vi "FileManager.vi"(6 "Function":enum16{"Switch", "Train"}(ring)=enum."Train", 8 "error in":errorcluster, 11 "file path":path=path "D:/Minecraft/mmc-stable-win32/MultiMC/instances/TRAINS 3-/.minecraft/saves/trains/opencomputers/442cd0d6-e139-46e7-881b-600456d36bc7/home") -> (0 "error out":errorcluster, 1 "SwitchDataArray":T1(array[cluster]), 2 "PathArray":path[](array[path]), 3 "TrainDataArray":T2(array[cluster]), 5 "RootPathArray":path[](array[path]))   [LabVIEW 2014]
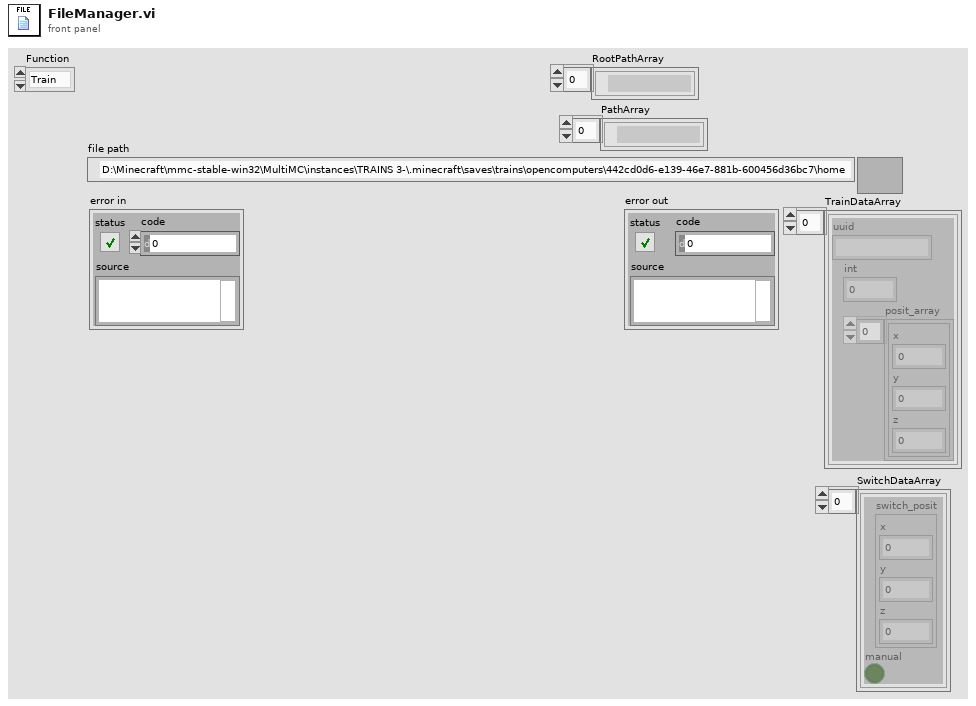
[diagram p1: front panel]
types:
  T1 = cluster{"switch_posit":cluster{"x":dbl, "y":dbl, "z":dbl}, "manual":bool}[]
  T2 = cluster{"uuid":string, "int":i32, "posit_array":cluster{"x":dbl, "y":dbl, "z":dbl}[]}[]
  T3 = cluster{"uuid":string, "int":i32, "posit_array":cluster{"x":dbl, "y":dbl, "z":dbl}[]}
  T4 = enum16{"open", "replace", "create", "open or create", "replace or create", "replace or create with confirmation"}
  T5 = cluster{"switch_posit":cluster{"x":dbl, "y":dbl, "z":dbl}, "manual":bool}
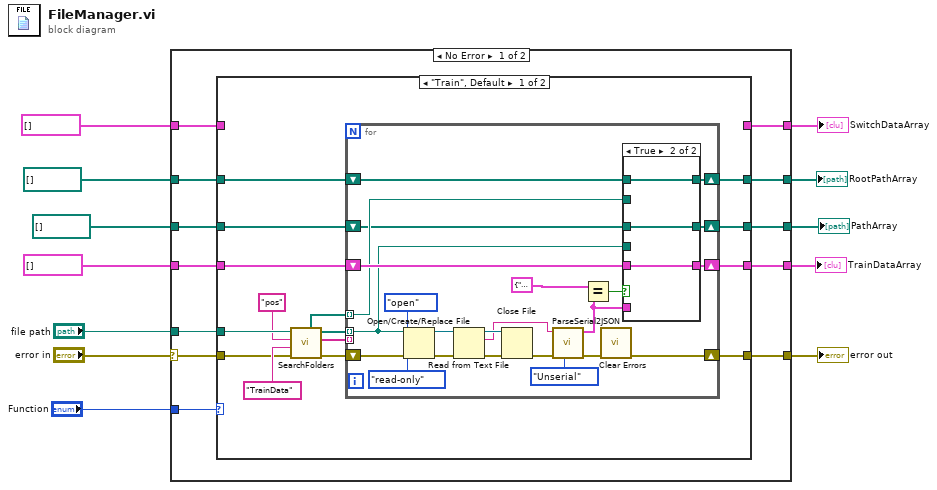
[diagram p0: block diagram]
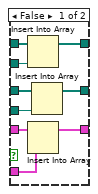
[diagram p2: hidden frame]
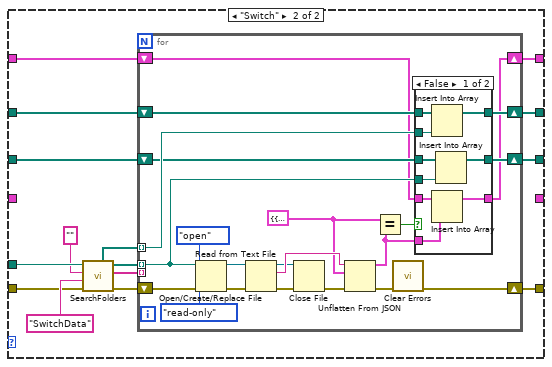
[diagram p3: hidden frame]
diagram:
  n1 = case shown="No Error" "error in" {
    selector: "error in" -> [w20 w128]
    tunnel: "file path" -> [w24 _]
    tunnel: [w23 w128] -> w11
    tunnel: T2 [] ("train_data_array") -> [w22 w127]
    tunnel: [w21 w127] -> w9
    tunnel: [w19 w126] -> w7
    tunnel: path[] [] -> [w18 w126]
    tunnel: [w16 w125] -> w4
    tunnel: path[] [] -> [w17 w125]
    tunnel: "Function" -> [w15 _]
    tunnel: T1 [] ("train_data_array") -> [w14 w124]
    tunnel: [w13 w124] -> w1
    frame No Error {
      n2 = case shown="\"Train\", Default" w15 {
        tunnel: w24 -> [w37 w87]
        tunnel: [w36 w86] -> w23
        tunnel: w22 -> [w32 _]
        tunnel: [w31 _] -> w21
        tunnel: w20 -> [w30 w82]
        tunnel: [w28 w80] -> w19
        tunnel: w18 -> [w27 w79]
        tunnel: w17 -> [w26 w78]
        tunnel: [w25 w77] -> w16
        tunnel: w14 -> [_ w76]
        tunnel: [_ w75] -> w13
        frame "Train", Default {
          n3 = call "SearchFolders.vi"("error in"=w30, "Folder"="TrainData", "regular expression"="pos", "file path"=w37) -> ("error out"=w38:errorcluster, "File Array"=w33:string[], "Path Array"=w39:path[], "Root Path Array"=w29:path[])  [unwired: 4 in]
          n4 = for {
            tunnel: w39 -> [w45] mode=indexing
            shift-right: [w57] -> w36
            shift-left: w38 -> [w60]
            tunnel: w33 -> [_] mode=indexing
            tunnel: w29 -> [w50] mode=indexing
            shift-right: [w51] -> w31
            shift-left: w32 -> [w53]
            shift-right: [w48] -> w28
            shift-left: w27 -> [w49]
            shift-right: [w47] -> w25
            shift-left: w26 -> [w46]
            n5 = Open/Create/Replace File(file path (use dialog)=w45, error in=w60, operation (0:open)=T4."open", access (0:read/write)=enum16{"read/write", "read-only", "write-only"}."read-only") -> (refnum out=w58:refnum<file>, error out=w59:errorcluster)  [unwired: 2 in, 1 out]
            n6 = Read from Text File(file (use dialog)=w58, error in=w59) -> (refnum out=w55:refnum<file>, text=w44:string, error out=w56:errorcluster)  [unwired: 2 in, 1 out]
            n7 = Close File(refnum=w55, error in=w56) -> (error out=w43:errorcluster)  [unwired: 1 out]
            n8 = call "ParseSerial2JSON.vi"("Function"=enum16{"Serial", "Unserial"}."Unserial", "error in (no error)"=w43, "input"=w44) -> ("error out"=w41:errorcluster, "output"=w42:T3)  [unwired: 6 in, 1 out]
            n9 = Equal?(x=T3 {"uuid"="", "int"=0, "posit_array"=[]} ("train_data"), y=w42) -> (x = y?=w52:bool)
            n10 = call <vilib>:"Clear Errors.vi"("error in (no error)"=w41) -> ("error out"=w57:errorcluster)  [unwired: 5 in, 1 out]
            n11 = case shown="True" w52 {
              tunnel: w53 -> [w71 w74]
              tunnel: w42 -> [w69 _]
              tunnel: [w70 w74] -> w51
              tunnel: w50 -> [w68 _]
              tunnel: w49 -> [w67 w73]
              tunnel: [w66 w73] -> w48
              tunnel: w46 -> [w65 w72]
              tunnel: [w64 w72] -> w47
              tunnel: w45 -> [w63 _]
              frame False {
                n12 = Insert Into Array(array=w67, new element=w68) -> (w66:path[])  [unwired: 1 in]
                n13 = Insert Into Array(array=w71, new element=w69) -> (w70:T2)  [unwired: 1 in]
                n14 = Insert Into Array(array=w65, new element=w63) -> (w64:path[])  [unwired: 1 in]
              }
              frame True {
              }
            }
          }
        }
        frame "Switch" {
          n15 = call "SearchFolders.vi"("error in"=w82, "Folder"="SwitchData", "regular expression"="", "file path"=w87) -> ("error out"=w88:errorcluster, "File Array"=w83:string[], "Path Array"=w89:path[], "Root Path Array"=w81:path[])  [unwired: 4 in]
          n16 = for {
            tunnel: w89 -> [w93] mode=indexing
            shift-right: [w105] -> w86
            shift-left: w88 -> [w109]
            tunnel: w83 -> [_] mode=indexing
            tunnel: w81 -> [w98] mode=indexing
            shift-right: [w96] -> w80
            shift-left: w79 -> [w97]
            shift-right: [w95] -> w77
            shift-left: w78 -> [w94]
            shift-right: [w91] -> w75
            shift-left: w76 -> [w92]
            w90 = T5 {"switch_posit"={"x"=0.0, "y"=0.0, "z"=0.0}, "manual"=FALSE} ("switch_data")
            n17 = Open/Create/Replace File(file path (use dialog)=w93, error in=w109, operation (0:open)=T4."open", access (0:read/write)=enum16{"read/write", "read-only", "write-only"}."read-only") -> (refnum out=w107:refnum<file>, error out=w108:errorcluster)  [unwired: 2 in, 1 out]
            n18 = Read from Text File(file (use dialog)=w107, error in=w108) -> (refnum out=w102:refnum<file>, text=w106:string, error out=w103:errorcluster)  [unwired: 2 in, 1 out]
            n19 = Close File(refnum=w102, error in=w103) -> (error out=w101:errorcluster)  [unwired: 1 out]
            n20 = Unflatten From JSON(JSON string=w106, type and defaults=w90, error in (no error)=w101) -> (value=w99:T5, error out=w104:errorcluster)  [unwired: 4 in]
            n21 = Equal?(x=w90, y=w99) -> (x = y?=w100:bool)
            n22 = call <vilib>:"Clear Errors.vi"("error in (no error)"=w104) -> ("error out"=w105:errorcluster)  [unwired: 5 in, 1 out]
            n23 = case shown="False" w100 {
              tunnel: w92 -> [w120 w123]
              tunnel: w99 -> [w118 _]
              tunnel: [w119 w123] -> w91
              tunnel: w98 -> [w117 _]
              tunnel: w97 -> [w116 w122]
              tunnel: [w115 w122] -> w96
              tunnel: w94 -> [w114 w121]
              tunnel: [w113 w121] -> w95
              tunnel: w93 -> [w112 _]
              frame False {
                n24 = Insert Into Array(array=w116, new element=w117) -> (w115:path[])  [unwired: 1 in]
                n25 = Insert Into Array(array=w120, new element=w118) -> (w119:T1)  [unwired: 1 in]
                n26 = Insert Into Array(array=w114, new element=w112) -> (w113:path[])  [unwired: 1 in]
              }
              frame True {
              }
            }
          }
        }
      }
    }
    frame Error {
    }
  }
  "error out" <- w11
  "TrainDataArray" <- w9
  "RootPathArray" <- w7
  "PathArray" <- w4
  "SwitchDataArray" <- w1
